vi "Tektronix DPO MSO 2000 4000 Series Acquire Multiple Digital Waveforms Example.vi"() -> ()   [LabVIEW 2017]
doc: "This example illustrates how to use autosetup and acquire multiple waveforms on multiple digital channels using the following steps:\n\n1. Specify a valid VISA session. \n2. Specify digital channels to be acquired.\n3. Specify a time-out value for reading waveform.\n4. Run the VI. The graph displays the waveforms you acquire. \n\n<B>Note:</B>\n-This VI does not work with DPO series oscilloscopes.\n- LabVIEW versions higher than 7.1 might display the data differently."
uses:
  <instrlib>/Tektronix DPO MSO 2000 4000 Series/Public/Data/Read (Multiple Digital Waveforms).vi
  <instrlib>/Tektronix DPO MSO 2000 4000 Series/Tektronix DPO MSO 2000 4000 Series.lvlib
panel:
  out "Digital Waveform Graph":digitalwaveform[](graph)
  in  "Digital Channels":u16[](array[ring])=[14] items=["Digital Channel D0"=14, "Digital Channel D1"=15, "Digital Channel D2"=16, "Digital Channel D3"=17, "Digital Channel D4"=18, "Digital Channel D5"=19, "Digital Channel D6"=20, "Digital Channel D7"=21, "Digital Channel D8"=22, "Digital Channel D9"=23, "Digital Channel D10"=24, "Digital Channel D11"=25, "Digital Channel D12"=26, "Digital Channel D13"=27, "Digital Channel D14"=28, "Digital Channel D15"=29]
  in  "Maximum Time (100000ms)":u32=100000
  in  "VISA Resource Name":refnum<visa-resource-name>
  # "(C) 2006 - 2016. National Instruments Corporation. ALL RIGHTS RESERVED."
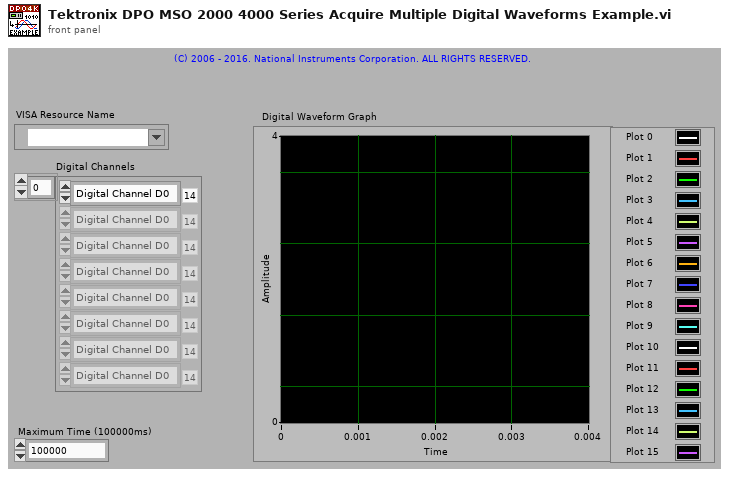
[diagram p1: front panel]
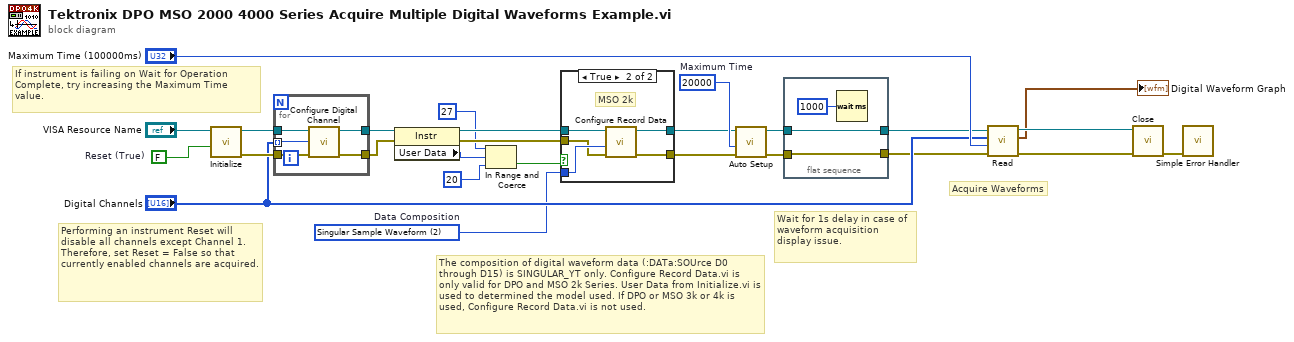
[diagram p0: block diagram]
diagram:
  w13 = u16 2 items=["Composite Sample Waveform", "Composite Peak Detect Waveform", "Singular Sample Waveform"]  # Data Composition
  w18 = u32 20000  # Maximum Time
  w22 = FALSE  # Reset (True)
  # "Wait for 1s delay in case of waveform acquisition display issue."
  # "The composition of digital waveform data (:DATa:SOUrce D0 through D15) is SINGULAR_YT only. Configure Record Data.vi is only valid for DPO and MSO 2k Series. User Data from Initialize.vi is used to determined the model used. If DPO or MSO 3k or 4k is used, Configure Record Data.vi is not used."
  # "Acquire Waveforms"
  # "If instrument is failing on Wait for Operation Complete, try increasing the Maximum Time value."
  # "Performing an instrument Reset will disable all channels except Channel 1. Therefore, set Reset = False so that currently enabled channels are acquired."
  n1 = call <instrlib>:"Initialize.vi"("Reset (True)"=w22, "VISA resource name"="VISA Resource Name") -> ("error out"=w20:errorcluster, "VISA resource name out"=w21:refnum<visa-resource-name>)  [unwired: 8 in]
  n2 = for {
    tunnel: w21 -> [w31]
    tunnel: w20 -> [w30]
    tunnel: [w29] -> w12
    tunnel: [w28] -> w11
    tunnel: "Digital Channels" -> [w27] mode=indexing
    n3 = call <instrlib>:"Configure Digital Channel.vi"("error in (no error)"=w30, "Digital Channel (14: Digital Channel 0)"=w27, "VISA resource name"=w31) -> ("error out"=w28:errorcluster, "VISA resource name out"=w29:refnum<visa-resource-name>)  [unwired: 7 in]
  }
  n4 = property class="Instr"(reference=w12, error in=w11) -> (reference out=w10:refnum<visa-resource-name>, error out=w9:errorcluster, "User Data"=w8:u32)
  n5 = In Range and Coerce(upper limit=u32 27, x=w8, lower limit=u32 20) -> (In Range?=w5:bool)  [unwired: 1 out]
  n6 = case shown="True" w5 {
    tunnel: [w33 w38] -> w15
    tunnel: [w32 w37] -> w14
    tunnel: w13 -> [_ w36]
    tunnel: w10 -> [w33 w35]
    tunnel: w9 -> [w32 w34]
    frame False {
      # "MSO 4k"
    }
    frame True {
      # "MSO 2k"
      n7 = call <instrlib>:"Configure Record Data.vi"("error in (no error)"=w34, "Data Composition (0: Composite Sample Waveform)"=w36, "VISA resource name"=w35) -> ("error out"=w37:errorcluster, "VISA resource name out"=w38:refnum<visa-resource-name>)  [unwired: 7 in]
    }
  }
  n8 = call <instrlib>:"Auto Setup.vi"("error in (no error)"=w14, "Maximum Time (10000ms)"=w18, "VISA resource name"=w15) -> ("error out"=w3:errorcluster, "VISA resource name out"=w4:refnum<visa-resource-name>)  [unwired: 7 in]
  n9 = flat-sequence {
    tunnel: w4 -> [w41]
    tunnel: [w41] -> w2
    tunnel: [w40] -> w1
    tunnel: w3 -> [w40]
    frame #0 {
      n10 = Wait (ms)(milliseconds to wait=u32 1000) -> ()  [unwired: 1 out]
    }
  }
  n11 = call-poly <instrlib>:"Read.vi"("error in (no error)"=w1, "Maximum Time (10000ms)"="Maximum Time (100000ms)", "Digital Channels"="Digital Channels", "VISA resource name"=w2) -> ("error out"=w23:errorcluster, "Digital Waveform Graph"=→"Digital Waveform Graph":digitalwaveform[], "VISA resource name out"=w24:refnum<visa-resource-name>)  [unwired: 5 in]
  n12 = call <instrlib>:"Close.vi"("error in (no error)"=w23, "VISA resource name"=w24) -> ("error out"=w25:errorcluster)  [unwired: 9 in]
  n13 = call <vilib>:"Simple Error Handler.vi"("error in (no error)"=w25) -> ()  [unwired: 4 in, 5 out]
